vi "Clean Up View.vi"(8 "error in (no error)":errorcluster, 11 "Message Queues in":T1) -> (0 "error out":errorcluster, 3 "dup Message Queues":T1)   [LabVIEW 2023, in "Weather Monitor Views.lvlib"]
doc: "Cleans up the message queues after a view has closed."
uses:
  Weather Monitor Views.lvlib
  support/Message Queue/All Message Queues.ctl
  support/Message Queue/Message Cluster.ctl
  support/Message Queue/Weather Message Queue.lvlib
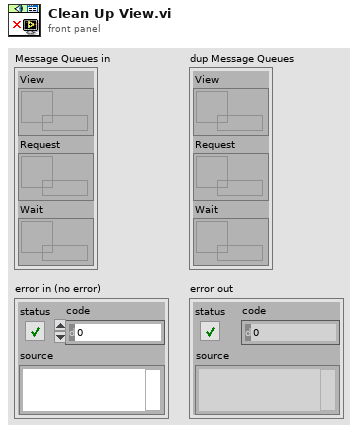
[diagram p1: front panel]
types:
  T1 = typedef "Weather Message Queue.lvlib/All Message Queues.ctl" = cluster{"View":refnum<queue>, "Request":refnum<queue>, "Wait":refnum<queue>}
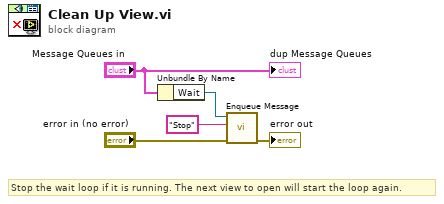
[diagram p0: block diagram]
diagram:
  # "Stop the wait loop if it is running. The next view to open will start the loop again."
  n1 = Unbundle By Name("Message Queues in") -> ("Wait"=w5:refnum<queue>)
  n2 = call "Enqueue Message.vi"("error in (no error)"="error in (no error)", "Message"="Stop", "Message Queue"=w5) -> ("error out"=→"error out":errorcluster)  [unwired: 7 in, 1 out]
  "dup Message Queues" <- "Message Queues in"
